vi "read_courbe.vi"() -> (1 "XY Plot Matrix":cluster{"all rows":dbl[], "all rows":dbl[]}(graph), 2 "error out":errorcluster)   [LabVIEW 2021]
uses:
  <vilib>/Utility/file.llb/Read Delimited Spreadsheet (DBL).vi
panel:
  out "new file path (Not A Path if cancelled)":path
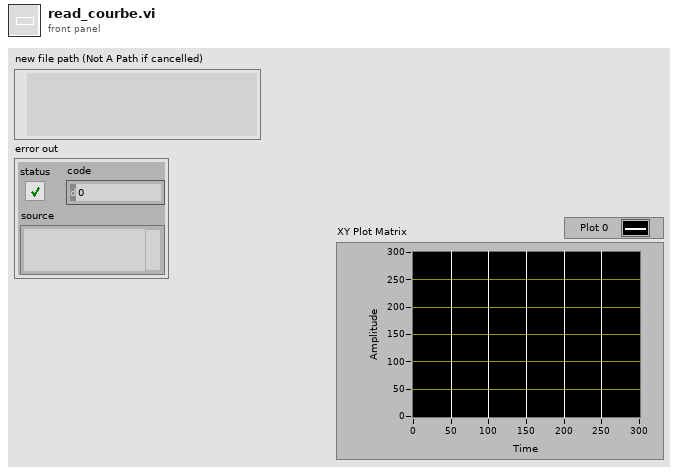
[diagram p1: front panel]
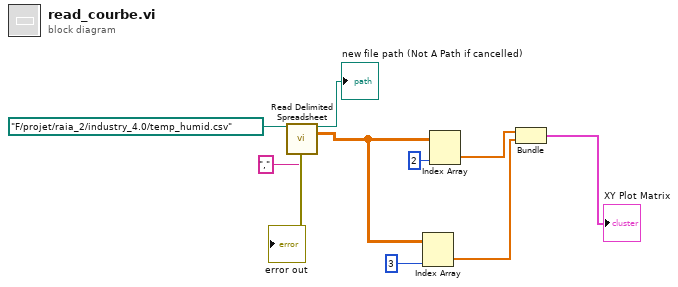
[diagram p0: block diagram]
diagram:
  n1 = call-poly <vilib>:"Read Delimited Spreadsheet.vi"("file path (dialog if empty)"=path "F:/projet/raia_2/industry_4.0/temp_humid.csv", "delimiter (\\t)"="," ("delimiter (\\t)")) -> ("new file path (Not A Path if cancelled)"=→"new file path (Not A Path if cancelled)":path, "all rows"=w3:dbl[][], "error out"=→"error out":errorcluster)  [unwired: 8 in, 3 out]
  n2 = Index Array(array=w3, index (col)=3) -> (element=w2:dbl[])  [unwired: 1 in]
  n3 = Index Array(array=w3, index (col)=2 ("disabled index (col)")) -> (element=w6:dbl[])  [unwired: 1 in]
  n4 = Bundle("all rows"=w6, "all rows"=w2) -> (→"XY Plot Matrix":cluster{"all rows":dbl[], "all rows":dbl[]})  [unwired: 1 in]
